vi "Configure Control Relay.vi"(0 "VISA resource name":refnum<visa-resource-name>, 1 "Unit No. (0)":i32 min=0 max=6, 4 "Module No.(0)":i32 min=0 max=9, 5 "DO No.(1)":i32=1 min=1 max=2, 7 "error in (no error)":errorcluster, 8 "Output Type":u16(ring) items=["Contact Output within Module", "Alarm", "Manual"], 9 "Selected Loop":u16(ring) items=["LOOP1", "LOOP2", "COMMON"], 10 "Relay Action on Alarm ACK":u16(ring) items=["Normal", "Reset"], 11 "Relay Deactivated Interval":u16(ring) items=["500ms", "1s", "2s"], 14 "Target Status":u16(ring) items=["Off", "ALARM1_OUT_LOOP1", "ALARM2_OUT_LOOP1", "ALARM3_OUT_LOOP1", "ALARM4_OUT_LOOP1", "ALARM1_LOOP1", "ALARM2_LOOP1", "ALARM3_LOOP1", "ALARM4_LOOP1", "STOP_RUN_LOOP1", "AUTO_MAN_LOOP1", "REMOTE_LOCAL_LOOP1", "AUTO_TUNNING_LOOP1", "EXPV_LOCALPV_LOOP1", "ALARM1_OUT_LOOP2", "ALARM2_OUT_LOOP2", "ALARM3_OUT_LOOP2", "ALARM4_OUT_LOOP2", "ALARM1_LOOP2", "ALARM2_LOOP2", "ALARM3_LOOP2", "ALARM4_LOOP2", "STOP_RUN_LOOP2", "AUTO_MAN_LOOP2", "AUTO_LOOP2", "MAN_LOOP2", "CASCADE_LOOP2", "REMOTE_LOCAL_LOOP2", "AUTO_TUNNING_LOOP2", "EXPV_LOCALPV_LOOP2", "DI1", "DI2", "DI3", "DI4", "DI5", "DI6", "DI7", "DI8", "AI1_BURNOUT", "AI1_ADERROR", "AI2_BURNOUT", "AI2_BURNOUT"], 15 "Energize_DeEnergize":u16(ring) items=["Energize", "De_Energize"], 16 "Alarm Action-Operation Mode":u16(ring) items=["And", "Or", "Reflash"], 17 "Alarm Action-Hold/NonHold":u16(ring) items=["Hold", "Nonhold"]) -> (20 "VISA resource name out":refnum<visa-resource-name>, 21 "DO No.":i32, 24 "Unit No.":i32, 25 "Module No.":i32, 27 "error out":errorcluster)   [LabVIEW 2020, in "Yokogawa GX Series.lvlib"]
doc: "Set Relay Actions\n\nCommand: SCtrlRelay"
uses:
  <instrlib>/Yokogawa GX Series/Yokogawa GX Series.lvlib
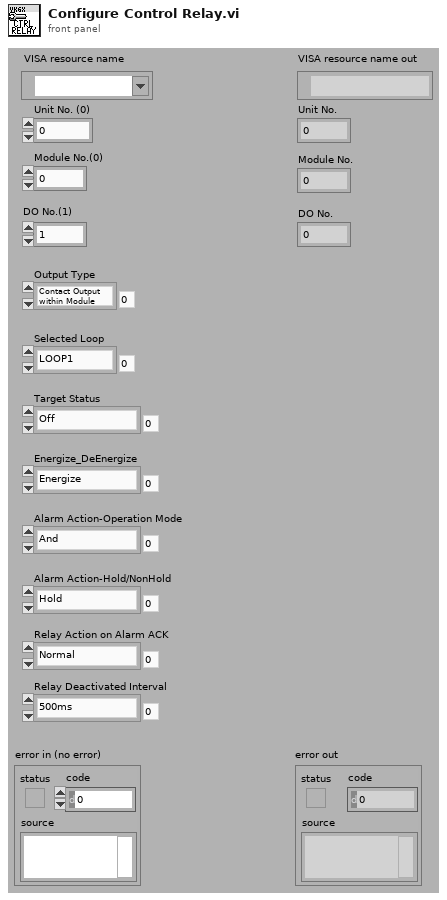
[diagram p1: front panel]
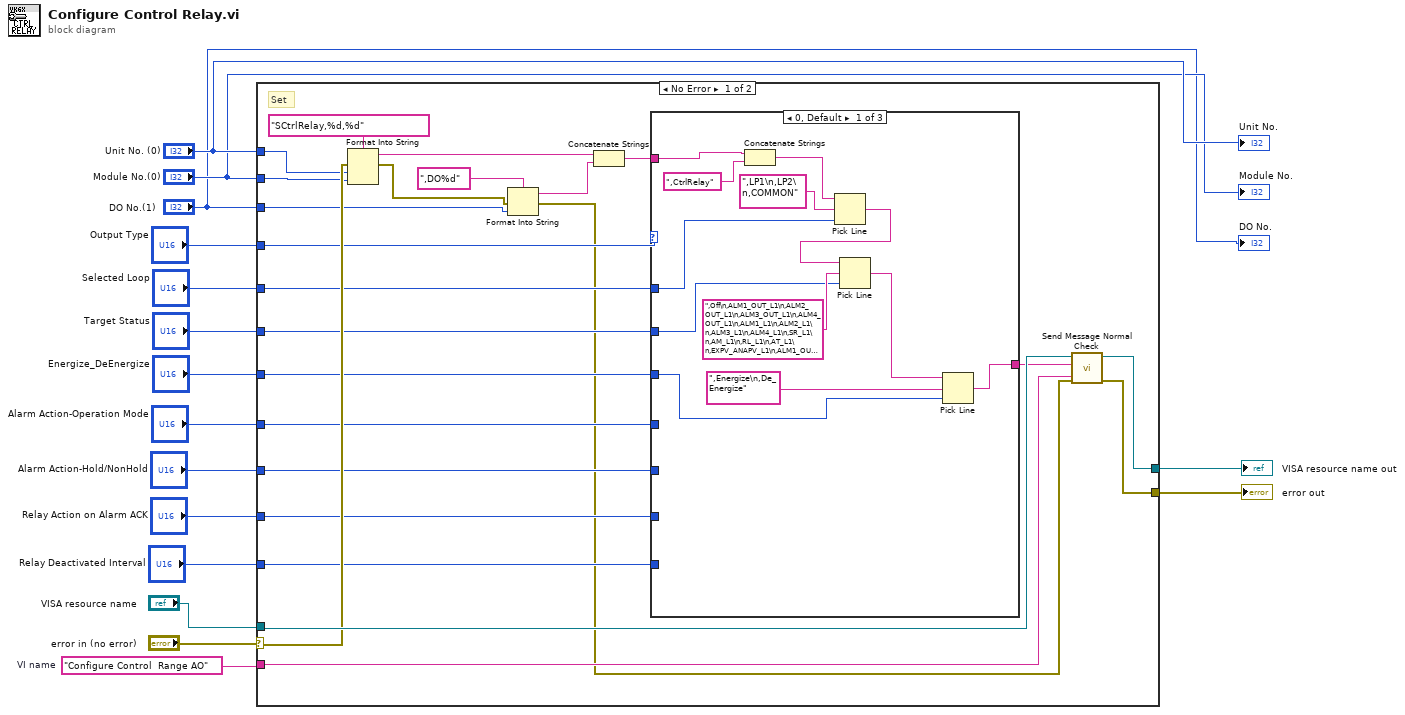
[diagram p0: block diagram]
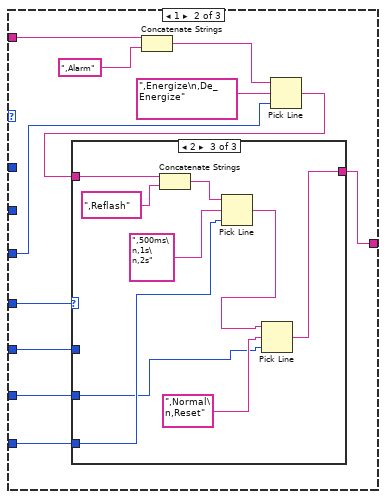
[diagram p2: hidden frame]
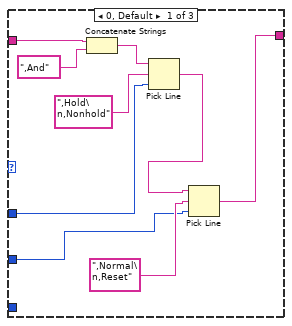
[diagram p3: hidden frame]
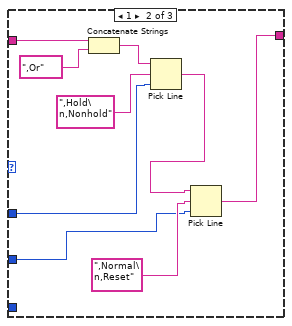
[diagram p4: hidden frame]
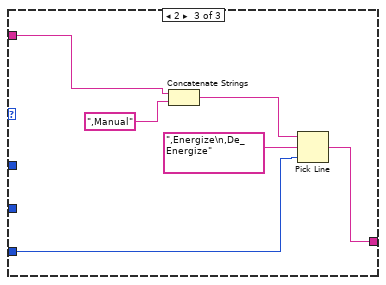
[diagram p5: hidden frame]
diagram:
  w12 = "Configure Control  Range AO"  # VI name
  n1 = case shown="No Error" "error in (no error)" {
    selector: "error in (no error)" -> [w36 w97]
    tunnel: [w40 w98] -> w16
    tunnel: [w39 w97] -> w15
    tunnel: "VISA resource name" -> [w38 w98]
    tunnel: w12 -> [w35 _]
    tunnel: "Unit No. (0)" -> [w34 _]
    tunnel: "Module No.(0)" -> [w33 _]
    tunnel: "DO No.(1)" -> [w31 _]
    tunnel: "Output Type" -> [w27 _]
    tunnel: "Selected Loop" -> [w25 _]
    tunnel: "Target Status" -> [w24 _]
    tunnel: "Energize_DeEnergize" -> [w23 _]
    tunnel: "Alarm Action-Operation Mode" -> [w21 _]
    tunnel: "Alarm Action-Hold/NonHold" -> [w20 _]
    tunnel: "Relay Action on Alarm ACK" -> [w19 _]
    tunnel: "Relay Deactivated Interval" -> [w18 _]
    frame No Error {
      # "Set"
      n2 = Format Into String(format string="SCtrlRelay,%d,%d", error in=w36, w34, w33) -> (resulting string=w29:string, error out=w30:errorcluster)  [unwired: 1 in]
      n3 = Format Into String(format string=",DO%d", error in=w30, w31) -> (resulting string=w28:string, error out=w17:errorcluster)  [unwired: 1 in]
      n4 = Concatenate Strings(w29, w28) -> (w26:string)
      n5 = case shown="0, Default" w27 {
        tunnel: w26 -> [w52 w60 w93]
        tunnel: w25 -> [w48 _ _]
        tunnel: w24 -> [w45 _ _]
        tunnel: w23 -> [w42 w57 w91]
        tunnel: [w41 w54 w92] -> w22
        tunnel: w21 -> [_ w58 _]
        tunnel: w20 -> [_ w56 _]
        tunnel: w19 -> [_ w55 _]
        tunnel: w18 -> [_ w53 _]
        frame 0, Default {
          n6 = Concatenate Strings(w52, ",CtrlRelay") -> (w50:string)
          n7 = Pick Line(string ("")=w50, multi-line string=",LP1\n,LP2\n,COMMON", line index=w48) -> (output string=w47:string)
          n8 = Pick Line(string ("")=w47, multi-line string=",Off\n,ALM1_OUT_L1\n,ALM2_OUT_L1\n,ALM3_OUT_L1\n,ALM4_OUT_L1\n,ALM1_L1\n,ALM2_L1\n,ALM3_L1\n,ALM4_L1\n,SR_L1\n,AM_L1\n,RL_L1\n,AT_L1\n,EXPV_ANAPV_L1\n,ALM1_OUT_L2\n,ALM2_OUT_L2\n,ALM3_OUT_L2\n,ALM4_OUT_L2\n,ALM1_L2\n,ALM2_L2\n,ALM3_L2\n,ALM4_L2\n,SR_L2\n,AM_L2\n,AUTO_L2\n,MAN_L2\n,CAS_L2\n,RL_L2\n,AT_L2\n,EXPV_ANAPV_L2\n,DI1\n,DI2\n,DI3\n,DI4\n,DI5\n,DI6\n,DI7\n,DI8\n,AI1_BOUT\n,AI1_ADERR\n,AI2_BOUT\n,AI2_ADERR", line index=w45) -> (output string=w44:string)
          n9 = Pick Line(string ("")=w44, multi-line string=",Energize\n,De_Energize", line index=w42) -> (output string=w41:string)
        }
        frame 1 {
          n10 = Concatenate Strings(w60, ",Alarm") -> (w62:string)
          n11 = Pick Line(string ("")=w62, multi-line string=",Energize\n,De_Energize", line index=w57) -> (output string=w59:string)
          n12 = case shown="2" w58 {
            tunnel: w59 -> [w72 w76 w85]
            tunnel: w56 -> [w68 w75 _]
            tunnel: w55 -> [w65 w74 w82]
            tunnel: [w64 w73 w83] -> w54
            tunnel: w53 -> [_ _ w84]
            frame 0, Default {
              n13 = Concatenate Strings(w72, ",And") -> (w70:string)
              n14 = Pick Line(string ("")=w70, multi-line string=",Hold\n,Nonhold", line index=w68) -> (output string=w67:string)
              n15 = Pick Line(string ("")=w67, multi-line string=",Normal\n,Reset", line index=w65) -> (output string=w64:string)
            }
            frame 1 {
              n16 = Concatenate Strings(w76, ",Or") -> (w80:string)
              n17 = Pick Line(string ("")=w80, multi-line string=",Hold\n,Nonhold", line index=w75) -> (output string=w78:string)
              n18 = Pick Line(string ("")=w78, multi-line string=",Normal\n,Reset", line index=w74) -> (output string=w73:string)
            }
            frame 2 {
              n19 = Concatenate Strings(w85, ",Reflash") -> (w89:string)
              n20 = Pick Line(string ("")=w89, multi-line string=",500ms\n,1s\n,2s", line index=w84) -> (output string=w87:string)
              n21 = Pick Line(string ("")=w87, multi-line string=",Normal\n,Reset", line index=w82) -> (output string=w83:string)
            }
          }
        }
        frame 2 {
          n22 = Concatenate Strings(w93, ",Manual") -> (w95:string)
          n23 = Pick Line(string ("")=w95, multi-line string=",Energize\n,De_Energize", line index=w91) -> (output string=w92:string)
        }
      }
      n24 = call <instrlib>:"Send Message Normal Check.vi"("Source (\"\")"=w35, "error in (no error)"=w17, "Send Message (\"\")"=w22, "VISA resource name"=w38) -> ("error out"=w39:errorcluster, "VISA resource name out"=w40:refnum<visa-resource-name>)  [unwired: 2 in, 4 out]
    }
    frame Error {
    }
  }
  "error out" <- w15
  "VISA resource name out" <- w16
  "Unit No." <- "Unit No. (0)"
  "Module No." <- "Module No.(0)"
  "DO No." <- "DO No.(1)"
